vi "写入固件.vi"(6 "selected path":path, 7 "路径对话框":bool, 8 "错误输入":errorcluster, 10 "保留原配置":bool=TRUE, 11 "MB session in":refnum<class "MB_Master.lvclass">) -> (0 "error out":errorcluster, 3 "MB session out":refnum<class "MB_Master.lvclass">)   [LabVIEW 2016, in "斯坦道CODMn新电路板.lvlib"]
uses:
  <vilib>/Plasmionique/MB Master/MB_Master/MB_Master.lvclass
  <vilib>/NI/Progress Bar/Controls/Update Bar Actions.ctl
  <vilib>/NI/Progress Bar/Controls/Progress Bar Properties.ctl
  <vilib>/Plasmionique/MB Master/MB_Master_Serial/MB_Master_Serial.lvclass
  E:/Program Files (x86)/National Instruments/LabVIEW 2016/vi.lib/Plasmionique/MB Master/MB_Master/MB_Master.lvclass
  <vilib>/regexp/Match Regular Expression.xnode
  <vilib>/Plasmionique/MB Master/MB Master.lvlib
  <vilib>/NI/Progress Bar/Progress Bar.lvlib
panel:
  in  "引用选择":enum16{"MB引用", "自建引用"}(ring)
  in  "VISA Resource":refnum<visa-resource-name>
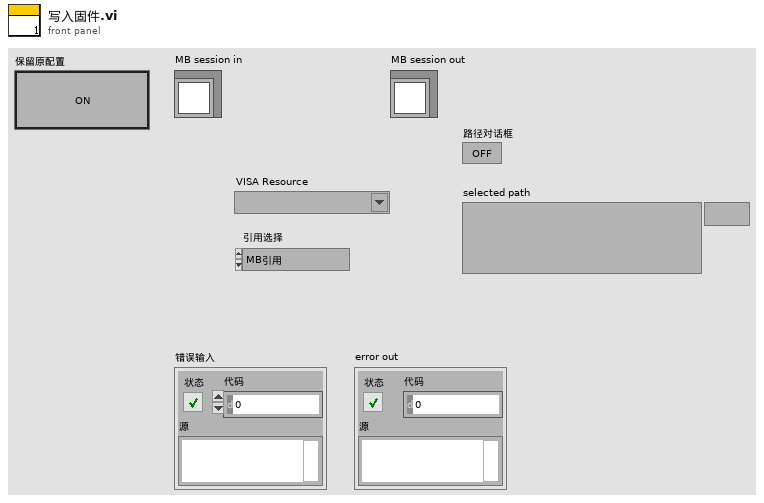
[diagram p1: front panel]
types:
  T1 = enum16{"open", "replace", "create", "open or create", "replace or create", "replace or create with confirmation"}
  T2 = enum16{"big-endian, network order", "native, host order", "little-endian"}
  T3 = typedef "Progress Bar.lvlib/Update Bar Actions.ctl" = enum16{"Add To Existing", "Set to Value"}
  T4 = cluster{"baud rate (bps)":u32, "stop bits":u16, "parity":u16, "flow control":u16, "timeout":u32, "retries":i32}
  T5 = typedef "Progress Bar.lvlib/Progress Bar Properties.ctl" = cluster{"Background Color":u32, "Installer Title":string, "Title Color":u32, "Action Text":string, "Text Color":u32, "Slider Value":u8, "Bar Color":u32, "Timeout":i32}
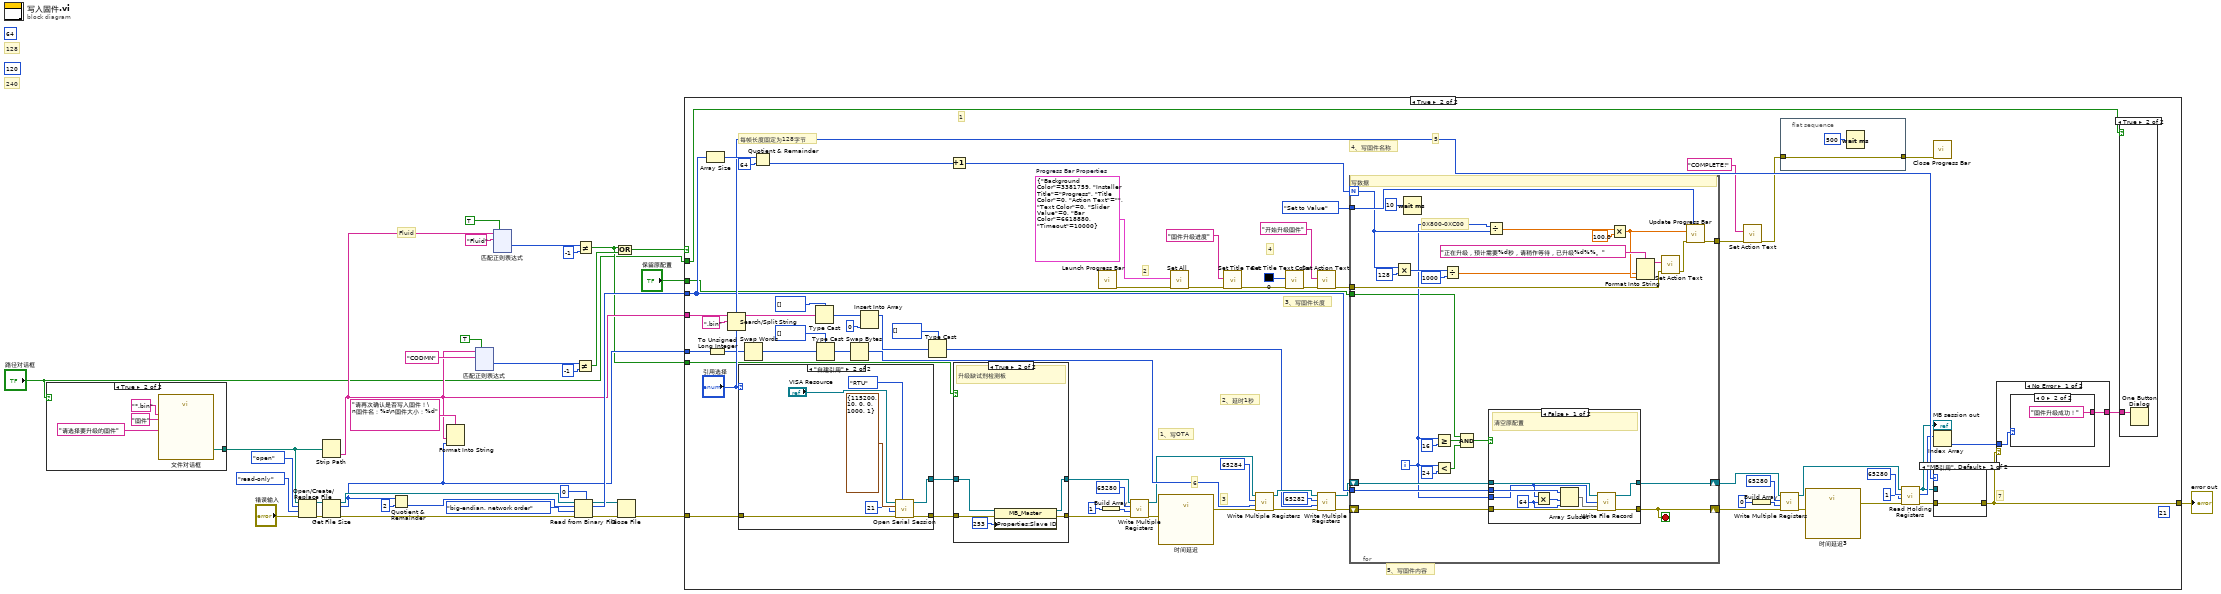
[diagram p0: block diagram]
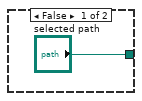
[diagram p2: hidden frame]
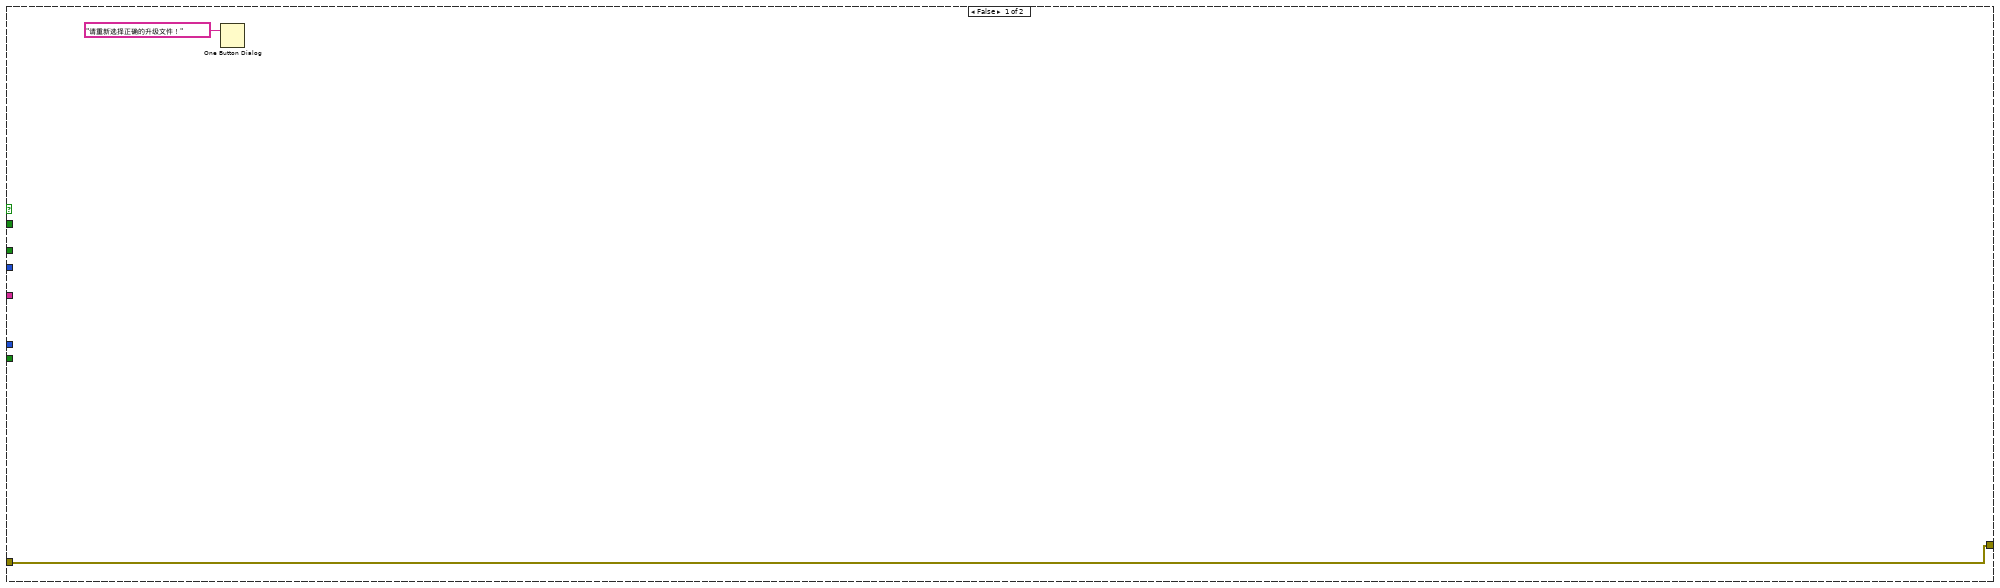
[diagram p3: hidden frame]
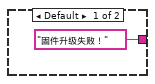
[diagram p6: hidden frame]
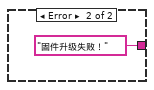
[diagram p7: hidden frame]
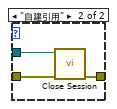
[diagram p8: hidden frame]
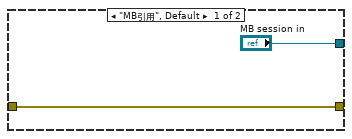
[diagram p9: hidden frame]
diagram:
  (unwired) 64 ("y")
  (unwired) 120 ("y")
  # "Fluid"
  # "240"
  # "128"
  n1 = case shown="True" "路径对话框" {
    tunnel: ["selected path" w36] -> w26
    frame False {
    }
    frame True {
      n2 = call "文件对话框"("prompt"="请选择要升级的固件", "pattern (all files)"="*.bin", "pattern label"="固件") -> ("selected path"=w36:path)  [unwired: 9 in, 3 out]
    }
  }
  n3 = Open/Create/Replace File(file path (use dialog)=w26, error in="错误输入", operation (0:open)=T1."open" ("操作(0:open)"), access (0:read/write)=enum16{"read/write", "read-only", "write-only"}."read-only" ("权限(0:read/write)")) -> (refnum out=w25:refnum<file>, error out=w23:errorcluster)  [unwired: 2 in, 1 out]
  n4 = Strip Path(path=w26) -> (name=w4:string)  [unwired: 1 out]
  n5 = Get File Size(file=w25, error in=w23) -> (refnum out=w24:refnum<file>, size (in bytes)=w18:i64, 0:w22:errorcluster)
  n6 = Quotient & Remainder(x=w18, y=i64 2) -> (floor(x/y)=w20:i64)  [unwired: 1 out]
  n7 = Format Into String(format string="请再次确认是否写入固件！\n固件名：%s\n固件大小：%d" ("格式字符串"), w4, w18) -> ()  [unwired: 2 in, 2 out]
  n8 = xnode "匹配正则表达式"("输入字符串"=w4, "正则表达式"="CODMN", "忽略大小写？(F)"=TRUE) -> ("匹配后偏移量"=w14:i32)  [unwired: 3 in, 4 out]
  n9 = xnode "匹配正则表达式"("输入字符串"=w4, "正则表达式"="Fluid", "忽略大小写？(F)"=TRUE) -> ("匹配后偏移量"=w7:i32)  [unwired: 3 in, 4 out]
  n10 = Read from Binary File(5:u16 0, 8:w22, 9:T2."big-endian, network order" ("字节顺序(0:big-endian, network order)"), 10:w20, 11:w24) -> (0:w11:errorcluster, 2:w19:u16[], 3:w12:refnum<file>)  [unwired: 1 in, 1 out]
  n11 = Not Equal?(x=w14, y=-1) -> (x != y?=w9:bool)
  n12 = Not Equal?(x=w7, y=-1) -> (x != y?=w2:bool)
  n13 = Or(x=w2, y=w9) -> (x .or. y?=w3:bool)
  n14 = Close File(refnum=w12, error in=w11) -> (error out=w10:errorcluster)  [unwired: 1 out]
  n15 = case shown="True" w3 {
    tunnel: w19 -> [_ w82]
    tunnel: w4 -> [_ w95]
    tunnel: w10 -> [w40 w96]
    tunnel: [w40 w79] -> w27
    tunnel: w18 -> [_ w84]
    tunnel: "保留原配置" -> [_ w52]
    tunnel: w2 -> [_ w49]
    tunnel: "路径对话框" -> [_ w41]
    frame False {
      n16 = One Button Dialog(message="请重新选择正确的升级文件！" ("消息")) -> ()  [unwired: 1 in, 1 out]
    }
    frame True {
      w76 = T5 {"Background Color"=3381759, "Installer Title"="Progress", "Title Color"=0, "Action Text"="", "Text Color"=0, "Slider Value"=0, "Bar Color"=6618880, "Timeout"=10000}  # Progress Bar Properties
      (unwired) 21 ("Value")
      # "7"
      # "6"
      # "5"
      # "4"
      # "3"
      # "2"
      # "1"
      # "每帧长度固定为128字节"
      # "5、写固件内容"
      # "4、写固件名称"
      # "3、写固件长度"
      # "2、延时1秒"
      # "1、写OTA"
      n17 = Array Size(array=w82) -> (size(s)=w110:i32)
      n18 = To Unsigned Long Integer(number=w84) -> (unsigned 32bit integer=w81:u32)
      n19 = Search/Split String(string=w95, search string/char (-)=".bin" ("搜索字符串/字符(-)")) -> (substring before match=w93:string)  [unwired: 1 in, 2 out]
      n20 = case shown="\"自建引用\"" "引用选择" {
        tunnel: ["MB session in" w138] -> w51
        tunnel: w96 -> [w132 w137]
        tunnel: [w132 w136] -> w48
        frame "MB引用", Default {
        }
        frame "自建引用" {
          n21 = call <vilib>:"Open Serial Session.vi"("Mode (RTU)"=enum16{"RTU", "ASCII"}."RTU", "Error in"=w137, "Slave ID"=u8 21, "Serial Config"=T4 {"baud rate (bps)"=115200, "stop bits"=10, "parity"=0, "flow control"=0, "timeout"=1000, "retries"=1}, "VISA Resource"="VISA Resource") -> ("Error out"=w136:errorcluster, "MB_Serial session"=w138:refnum<class "MB_Master_Serial.lvclass">)  [unwired: 5 in]
        }
      }
      n22 = Swap Words(1:w81) -> (0:w80:u32)
      n23 = Quotient & Remainder(x=w110, y=64) -> (floor(x/y)=w111:i32)  [unwired: 1 out]
      n24 = Type Cast(type=u8[] [], x=w93) -> (*(type *) &x=w43:u8[])
      n25 = Type Cast(type=u16[] [], x=w80) -> (*(type *) &x=w104:u16[])
      n26 = Swap Bytes(anything=w104) -> (byte swapped=w103:u16[])
      n27 = Insert Into Array(array=w43, new element=u8 0 ("新元素/子数组")) -> (w44:u8[])  [unwired: 1 in]
      n28 = Type Cast(type=u16[] [], x=w44) -> (*(type *) &x=w42:u16[])
      n29 = Increment(x=w111) -> (x+1=w83:i32)
      n30 = case shown="True" w49 {
        tunnel: w51 -> [w114 w119]
        tunnel: [w114 w118] -> w50
        tunnel: w48 -> [w113 w115]
        tunnel: [w113 w116] -> w47
        frame False {
          # "升级主板"
        }
        frame True {
          # "升级缺试剂检测板"
          n31 = property class="MB_Master"(reference=w119, error in=w115, "Properties:Slave ID"=u8 253 ("Slave ID")) -> (reference out=w118:refnum<class "MB_Master.lvclass">, error out=w116:errorcluster)
        }
      }
      n32 = call <vilib>:"Launch Progress Bar.vi"() -> ("error out"=w75:errorcluster)  [unwired: 10 in, 1 out]
      n33 = Build Array(u16 1 ("value")) -> (w97:u16[])
      n34 = call <vilib>:"Write Multiple Registers.vi"("error in (no error)"=w47, "values"=w97, "starting address"=u16 65280, "MB session in"=w50) -> ("error out"=w106:errorcluster, "MB session out"=w87:refnum<class "MB_Master.lvclass">)  [unwired: 6 in]
      n35 = call "时间延迟"("error in (no error)"=w106) -> ("error out"=w88:errorcluster)  [unwired: 10 in]
      n36 = call <vilib>:"Set All.vi"("error in (no error)"=w75, "Progress Bar Properties (Default)"=w76) -> ("error out"=w69:errorcluster)  [unwired: 9 in]
      n37 = call <vilib>:"Set Title Text.vi"("error in (no error)"=w69, "Installer Title"="固件升级进度") -> ("error out"=w67:errorcluster)  [unwired: 9 in]
      n38 = call <vilib>:"Write Multiple Registers.vi"("error in (no error)"=w88, "values"=w103, "starting address"=u16 65284, "MB session in"=w87) -> ("error out"=w101:errorcluster, "MB session out"=w102:refnum<class "MB_Master.lvclass">)  [unwired: 6 in]
      n39 = call <vilib>:"Set Title Text Color.vi"("error in (no error)"=w67, "Color Box"=u32 0) -> ("error out"=w70:errorcluster)  [unwired: 9 in]
      n40 = call <vilib>:"Set Action Text.vi"("error in (no error)"=w70, "Action Text"="开始升级固件") -> ("error out"=w64:errorcluster)  [unwired: 9 in]
      n41 = call <vilib>:"Write Multiple Registers.vi"("error in (no error)"=w101, "values"=w42, "starting address"=u16 65282, "MB session in"=w102) -> ("error out"=w61:errorcluster, "MB session out"=w62:refnum<class "MB_Master.lvclass">)  [unwired: 6 in]
      n42 = for {
        N: w83 -> [w149]
        shift-right: [w164] -> w57
        shift-left: w62 -> [w166]
        shift-right: [w140] -> w53
        shift-left: w61 -> [w165]
        tunnel: w82 -> [w162]
        tunnel: Update_Bar_Actions."Set to Value" ("Action") -> [w161]
        tunnel: w64 -> [w159]
        tunnel: [w160] -> w63
        tunnel: w52 -> [w141]
        i -> [w146]
        stop <- w140 stop-if-true
        # "0X800-0XC00"
        # "写数据"
        n43 = Multiply(x=w149, y=128) -> (x*y=w153:i32)
        n44 = Wait (ms)(milliseconds to wait=u32 10) -> ()  [unwired: 1 out]
        n45 = Greater Or Equal?(x=w146, y=16) -> (x >= y?=w144:bool)
        n46 = Less?(x=w146, y=24) -> (x < y?=w143:bool)
        n47 = Divide(x=w153, y=u32 1000) -> (x/y=w150:dbl)
        n48 = Compound Arithmetic op=AND ("复合运算")(w141, w144, w143) -> (w142:bool)
        n49 = Divide(x=w146, y=w149) -> (x/y=w155:dbl)
        n50 = case shown="False" w142 {
          tunnel: w166 -> [w175 w177]
          tunnel: w165 -> [w174 w176]
          tunnel: [w173 w177] -> w164
          tunnel: [w172 w176] -> w140
          tunnel: w162 -> [w171 _]
          tunnel: w146 -> [w167 _]
          frame False {
            w169 = 64 ("长度")
            # "清空原配置"
            n51 = Multiply(x=w167, y=w169) -> (x*y=w168:i32)
            n52 = Array Subset(array=w171, index=w168, length=w169) -> (w170:u16[])
            n53 = call "Write File Record.vi"("MB session in"=w175, "Record Number"=w167, "values"=w170, "error in (no error)"=w174) -> ("MB session out"=w173:refnum<class "MB_Master.lvclass">, "error out"=w172:errorcluster)  [unwired: 10 in]
          }
          frame True {
            # "保留原配置"
          }
        }
        n54 = Multiply(x=w155, y=100.0) -> (x*y=w151:dbl)
        n55 = Format Into String(format string="正在升级，预计需要%d秒，请稍作等待，已升级%d%%。" ("格式字符串"), w150, w151) -> (resulting string=w156:string)  [unwired: 2 in, 1 out]
        n56 = call <vilib>:"Set Action Text.vi"("error in (no error)"=w159, "Action Text"=w156) -> ("error out"=w158:errorcluster)  [unwired: 9 in]
        n57 = call <vilib>:"Update Progress Bar.vi"("Action"=w161, "error in (no error)"=w158, "Value"=w151) -> ("error out"=w160:errorcluster)  [unwired: 8 in]
      }
      n58 = call <vilib>:"Set Action Text.vi"("error in (no error)"=w63, "Action Text"="COMPLETE!") -> ("error out"=w72:errorcluster)  [unwired: 9 in]
      n59 = Build Array(0 ("value")) -> (w58:i32[])
      n60 = flat-sequence {
        tunnel: w72 -> [w120]
        tunnel: [w120] -> w74
        frame #0 {
          n61 = Wait (ms)(milliseconds to wait=u32 500) -> ()  [unwired: 1 out]
        }
      }
      n62 = call <vilib>:"Write Multiple Registers.vi"("error in (no error)"=w53, "values"=w58, "starting address"=u16 65280, "MB session in"=w57) -> ("error out"=w55:errorcluster, "MB session out"=w56:refnum<class "MB_Master.lvclass">)  [unwired: 6 in]
      n63 = call "时间延迟3"("error in (no error)"=w55) -> ("error out"=w54:errorcluster)  [unwired: 10 in]
      n64 = call <vilib>:"Read Holding Registers.vi"("error in (no error)"=w54, "quantity"=u16 1, "starting address"=u16 65280, "MB session in"=w56) -> ("error out"=w85:errorcluster, "Registers"=w89:u16[], "MB session out"=w86:refnum<class "MB_Master.lvclass">)  [unwired: 5 in]
      "MB session out" <- w86
      n65 = call <vilib>:"Close Progress Bar.vi"("error in (no error)"=w74) -> ()  [unwired: 9 in, 2 out]
      n66 = Index Array(array=w89) -> (element=w78:u16)  [unwired: 1 in]
      n67 = case shown="\"MB引用\", Default" "引用选择" {
        tunnel: w86 -> [_ w130]
        tunnel: w85 -> [w127 w129]
        tunnel: [w127 w128] -> w79
        frame "MB引用", Default {
        }
        frame "自建引用" {
          n68 = call-dynamic "Close Session.vi"("error in (no error)"=w129, "MB session in"=w130) -> ("error out"=w128:errorcluster)  [unwired: 9 in]
        }
      }
      n69 = case shown="No Error" w79 {
        tunnel: w78 -> [w123 _]
        tunnel: [w122 "固件升级失败！"] -> w77
        frame No Error {
          n70 = case shown="0" w123 {
            tunnel: ["固件升级失败！" "固件升级成功！"] -> w122
            frame Default {
            }
            frame 0 {
            }
          }
        }
        frame Error {
        }
      }
      n71 = case shown="True" w41 {
        tunnel: w77 -> [_ w112]
        frame False {
        }
        frame True {
          n72 = One Button Dialog(message=w112) -> ()  [unwired: 1 in, 1 out]
        }
      }
    }
  }
  "error out" <- w27
